vi "controls_to_2d_array.vi"(8 "error in (no error)":errorcluster, 11 "Controls[]":refnum<vi>[](array[refnum])) -> (3 "Array":string[][](array[string]))   [LabVIEW 2018]
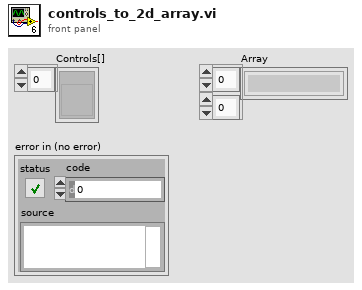
[diagram p1: front panel]
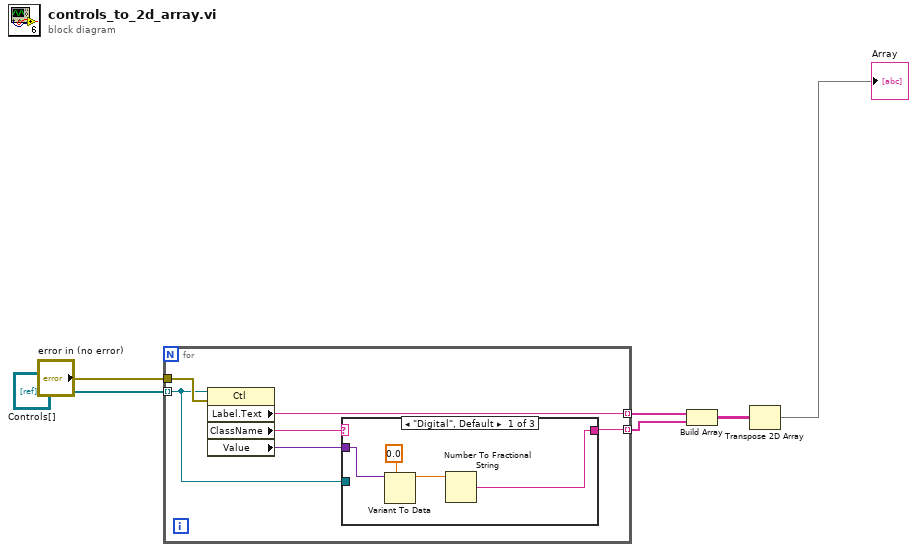
[diagram p0: block diagram]
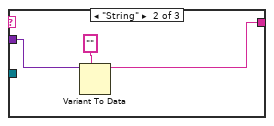
[diagram p2: hidden frame]
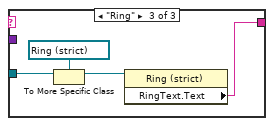
[diagram p3: hidden frame]
diagram:
  n1 = for {
    tunnel: "Controls[]" -> [w10] mode=indexing
    tunnel: "error in (no error)" -> [w12]
    tunnel: [w8] -> w3 mode=indexing
    tunnel: [w7] -> w4 mode=indexing
    n2 = property class="Ctl"(reference=w10, error in=w12) -> ("Label.Text"=w8:string, "ClassName"=w11:string, "Value"=w9:variant)  [unwired: 2 out]
    n3 = case shown="\"Digital\", Default" w11 {
      tunnel: w10 -> [_ _ w23]
      tunnel: w9 -> [w16 w19 _]
      tunnel: [w13 w17 w20] -> w7
      frame "Digital", Default {
        n4 = Variant To Data(type=0.0, Variant=w16) -> (data=w14:dbl)  [unwired: 1 in, 1 out]
        n5 = Number To Fractional String(number=w14) -> (F-format string=w13:string)  [unwired: 3 in]
      }
      frame "String" {
        n6 = Variant To Data(type="", Variant=w19) -> (data=w17:string)  [unwired: 1 in, 1 out]
      }
      frame "Ring" {
        n7 = To More Specific Class(target class=refnum<vi> refnum ("reference out"), reference=w23) -> (specific class reference=w21:refnum<vi>)  [unwired: 1 in, 1 out]
        n8 = property on="Property Node" class="Ring (strict)"(reference=w21) -> ("RingText.Text"=w20:string)  [unwired: 1 in, 2 out]
      }
    }
  }
  n9 = Build Array(w3, w4) -> (w5:string[][])
  n10 = Transpose 2D Array(2D array=w5) -> (transposed array=→"Array":string[][])
